vi "ExperimentDataEditor.vi"(11 "Experiment.lvclass":refnum<class "Experiment.lvclass">) -> ()   [LabVIEW 2012, in "Experiment.lvclass"]
uses:
  Experiment.lvclass
  DevicesClass/BaseDevice/BaseDevice.lvclass
panel:
  in  "Experiment.lvclass Out":refnum<class "Experiment.lvclass">
  in  "LoadedInst":i32
  in  "BaseDev Data":T1={"Nom de ressource VISA"="", "DeviceCtrl"=[], "DataNames"=[], "ScanParamOut"=0.0, "HeaderString"="", "Functions"=[], "ScanFunctionIndex"=0, "Function"="", "StartStatPanel"=FALSE, "PanelVIRef"=refnum, "SubPanelRef"=refnum, "SubPanelCtrl"=[], "LoadedPanelIndex"=-1, "InstrumentName"="", "AvailFuncPan"=["ClassPanel"], "ScanTable"=[], "ScanPanelRef"=refnum, "ScanPanelPath"=path "", "LastScanPos"=0.0, "Beforewait(ms)"=0, "Afterwait(ms)"=0, "SynchToClk(ms)"=-1, "FuncPanelIndex"=-1, "ClassQueue"=refnum, "ClassEvent"=refnum, "InstrParam"=[], "DatDisplayNm"=[], "ShowInstrNm"=[], "ShowParSuffix"=[], "ShowScanSuffix"=[], "ShowParValue"=[], "ParSuffix"=[], "ScanSuffix"=[]}
  in  "Experiment Data":T2
  in  "stop":bool
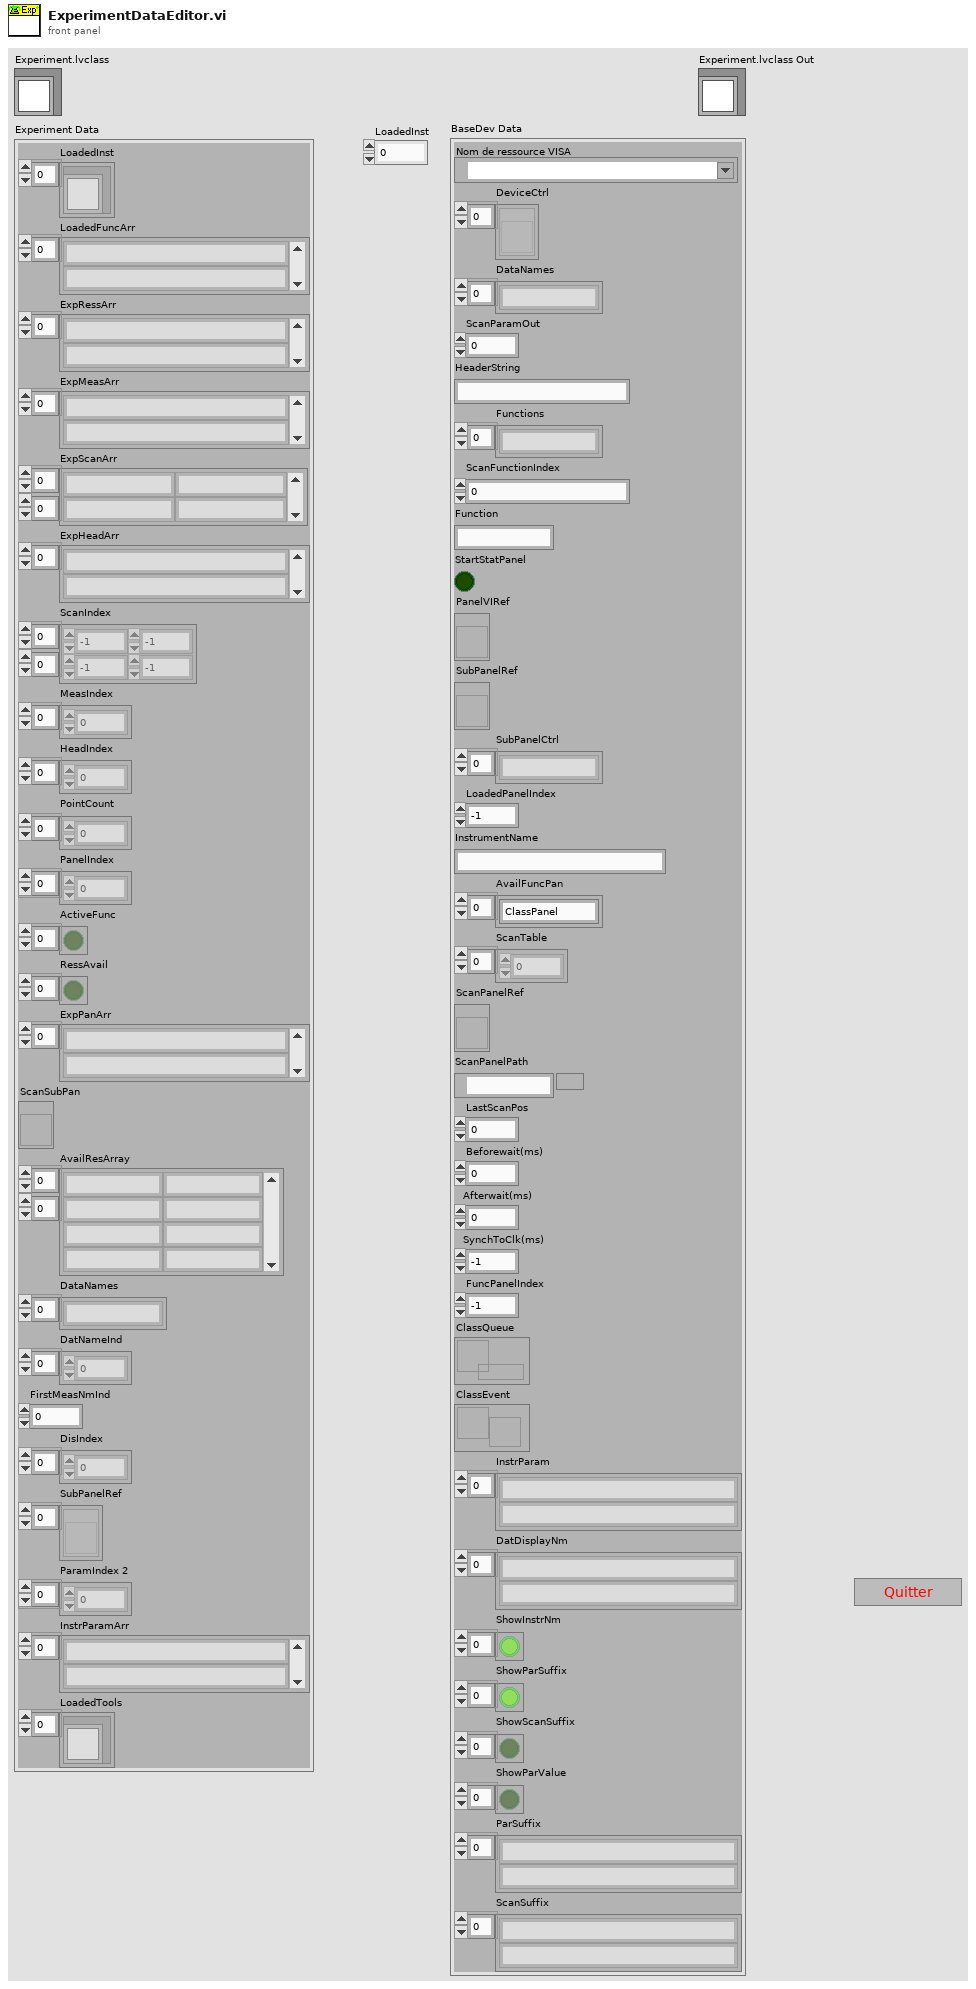
[diagram p1: front panel]
types:
  T1 = cluster{"Nom de ressource VISA":refnum<visa-resource-name>, "DeviceCtrl":refnum<vi>[], "DataNames":string[], "ScanParamOut":dbl, "HeaderString":string, "Functions":string[], "ScanFunctionIndex":i32, "Function":string, "StartStatPanel":bool, "PanelVIRef":refnum<vi>, "SubPanelRef":refnum<vi>, "SubPanelCtrl":string[], "LoadedPanelIndex":i32, "InstrumentName":string, "AvailFuncPan":string[], "ScanTable":dbl[], "ScanPanelRef":refnum<vi>, "ScanPanelPath":path, "LastScanPos":dbl, "Beforewait(ms)":u32, "Afterwait(ms)":u32, "SynchToClk(ms)":i32, "FuncPanelIndex":i32, "ClassQueue":refnum<queue>, "ClassEvent":refnum<user-event>, "InstrParam":string[], "DatDisplayNm":string[], "ShowInstrNm":bool[], "ShowParSuffix":bool[], "ShowScanSuffix":bool[], "ShowParValue":bool[], "ParSuffix":string[], "ScanSuffix":string[]}
  T2 = cluster{"LoadedInst":refnum<class "BaseDevice.lvclass">[], "LoadedFuncArr":string[], "ExpRessArr":string[], "ExpMeasArr":string[], "ExpScanArr":string[][], "ExpHeadArr":string[], "ScanIndex":i32[][], "MeasIndex":i32[], "HeadIndex":i32[], "PointCount":i32[], "PanelIndex":i32[], "ActiveFunc":bool[], "RessAvail":bool[], "ExpPanArr":string[], "ScanSubPan":refnum<vi>, "AvailResArray":string[][], "DataNames":string[], "DatNameInd":i32[], "FirstMeasNmInd":i32, "DisIndex":i32[], "SubPanelRef":refnum<vi>[], "ParamIndex 2":i32[], "InstrParamArr":string[], "LoadedTools":refnum<class "BaseDevice.lvclass">[]}
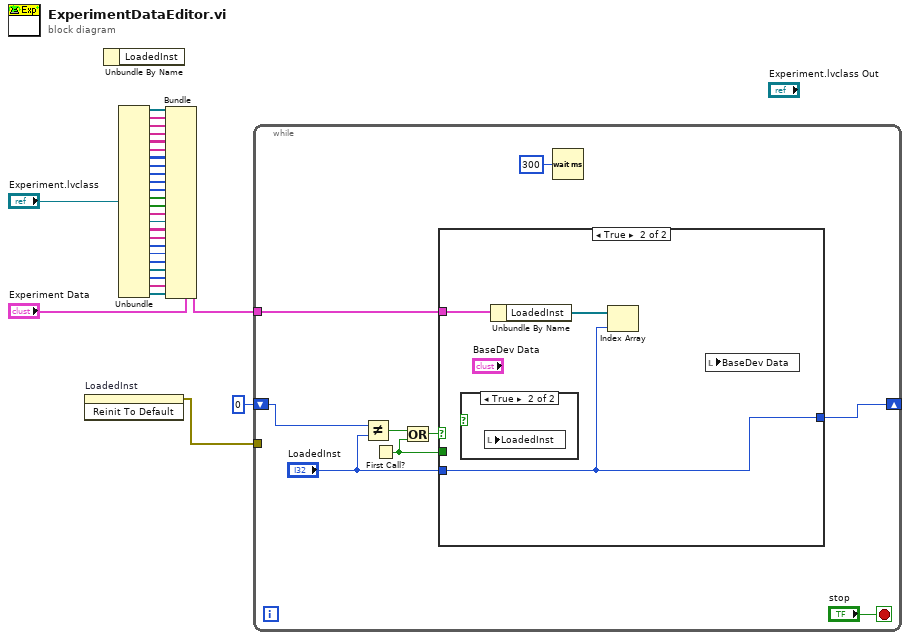
[diagram p0: block diagram]
diagram:
  n1 = invoke on="LoadedInst" class="DigNum (strict)" method="Reinit To Default"() -> (error out=w27:errorcluster)  [unwired: 3 in, 2 out]
  n2 = Unbundle By Name() -> ()  [unwired: 1 in, 1 out]
  n3 = Unbundle("Experiment.lvclass") -> (w24:refnum<class "BaseDevice.lvclass">[], w23:string[], w22:string[], w21:string[], w20:string[][], w19:string[], w18:i32[][], w17:i32[], w16:i32[], w15:i32[], w14:i32[], w13:bool[], w12:bool[], w11:string[], w10:refnum<vi>, w9:string[][], w8:string[], w7:i32[], w6:i32, w5:i32[], w4:refnum<vi>[], w3:i32[], w2:string[], w1:refnum<class "BaseDevice.lvclass">[])
  n4 = Bundle(cluster="Experiment Data", "LoadedInst"=w24, "LoadedFuncArr"=w23, "ExpRessArr"=w22, "ExpMeasArr"=w21, "ExpScanArr"=w20, "ExpHeadArr"=w19, "ScanIndex"=w18, "MeasIndex"=w17, "HeadIndex"=w16, "PointCount"=w15, "PanelIndex"=w14, "ActiveFunc"=w13, "RessAvail"=w12, "ExpPanArr"=w11, "ScanSubPan"=w10, "AvailResArray"=w9, "DataNames"=w8, "DatNameInd"=w7, "FirstMeasNmInd"=w6, "DisIndex"=w5, "SubPanelRef"=w4, "ParamIndex 2"=w3, "InstrParamArr"=w2, "LoadedTools"=w1) -> (w25:T2)
  n5 = while {
    shift-right: [w36] -> _
    shift-left: 0 ("LoadedInst") -> [w34]
    tunnel: w25 -> [w31]
    tunnel: w27 -> [_]
    stop <- "stop" stop-if-true
    n6 = Not Equal?(x=w34, y="LoadedInst") -> (x != y?=w33:bool)
    n7 = First Call?() -> (First Call?: T/F=w30:bool)
    n8 = Or(x=w33, y=w30) -> (x .or. y?=w32:bool)
    n9 = case shown="True" w32 {
      tunnel: [_ w39] -> w36
      tunnel: "LoadedInst" -> [_ w39]
      tunnel: w31 -> [_ w41]
      tunnel: w30 -> [_ _]
      frame False {
      }
      frame True {
        n10 = case shown="True" {
          selector: _ -> [_ _]
          frame False {
          }
          frame True {
            n11 = local read "LoadedInst"() -> ()  [unwired: 1 in]
          }
        }
        n12 = Unbundle By Name(w41) -> ("LoadedInst"=w40:refnum<class "BaseDevice.lvclass">[])
        n13 = Index Array(array=w40, index=w39) -> ()  [unwired: 1 out]
        n14 = local read "BaseDev Data"() -> ()  [unwired: 1 in]
      }
    }
    n15 = Wait (ms)(milliseconds to wait=u32 300) -> ()  [unwired: 1 out]
  }
